vi "Find One by Column.vi"(7 "Column Criteria":refnum<class "Type.lvclass">, 8 "error in (no error)":errorcluster, 9 "Entity Definition":refnum<class "Type.lvclass">[](array[class]), 10 "Table Name":string, 11 "Database in":refnum<class "SQLite.lvclass">) -> (0 "error out":errorcluster, 2 "Result Row":refnum<class "Result Row.lvclass">, 3 "Database out":refnum<class "SQLite.lvclass">)   [LabVIEW 2020, in "Conditum SQLite.lvlib" / "SQLite.lvclass"]
uses:
  SQLite.lvclass
  SQLite.lvclass/SQLite.ctl
  <vilib>/IlluminatedG/IG Conditum Base/Conditum/Columns/Type/Type.lvclass
  <vilib>/drjdpowell/SQLite Library/SQL Connection/Connection.lvclass
  <vilib>/IlluminatedG/IG Conditum Base/Conditum/Columns/ID/ID.lvclass
  <vilib>/drjdpowell/SQLite Library/SQL Statement/SQL Statement.lvclass
  <vilib>/IlluminatedG/IG Conditum Base/Conditum/Columns/Boolean/Boolean.lvclass
  <vilib>/IlluminatedG/IG Conditum Base/Conditum/Columns/Integer/Integer.lvclass
  <vilib>/IlluminatedG/IG Conditum Base/Conditum/Columns/Double/Double.lvclass
  <vilib>/IlluminatedG/IG Conditum Base/Conditum/Columns/Timestamp/Timestamp.lvclass
  <vilib>/IlluminatedG/IG Conditum Base/Conditum/Columns/String/String.lvclass
  <vilib>/IlluminatedG/IG Conditum Base/Conditum/Database Platform/Database Platform.lvclass
  C:/Program Files (x86)/National Instruments/LabVIEW 2020/vi.lib/IlluminatedG/IG Conditum Base/Conditum/Columns/Type/Type.lvclass
  C:/Program Files (x86)/National Instruments/LabVIEW 2020/vi.lib/IlluminatedG/IG Conditum Base/Conditum/Database Platform/Database Platform.lvclass
  <vilib>/IlluminatedG/IG Conditum Base/Conditum/Result Row/Result Row.lvclass
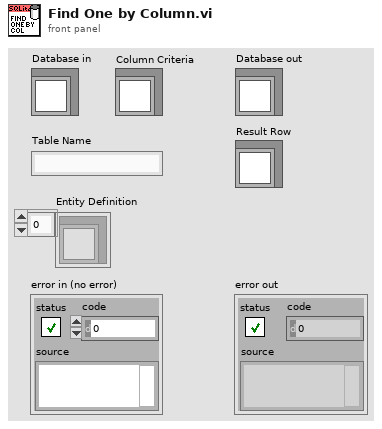
[diagram p1: front panel]
types:
  T1 = typedef "Conditum.lvlib/Field Type.ctl" = enum16{"None", "ID", "Boolean", "Integer", "Double", "Timestamp", "String", "Text", "Entity"}
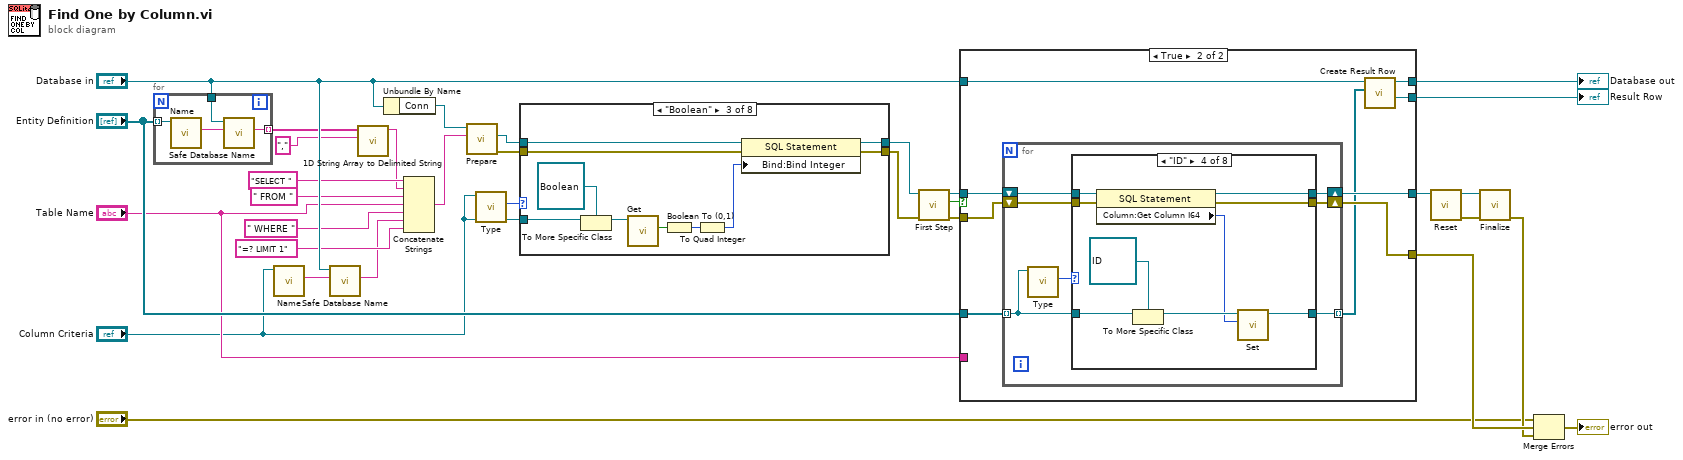
[diagram p0: block diagram]
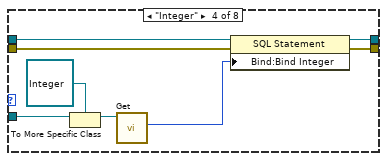
[diagram p4: hidden frame]
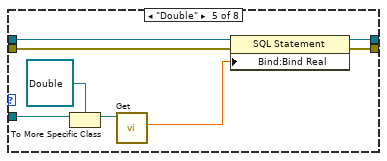
[diagram p5: hidden frame]
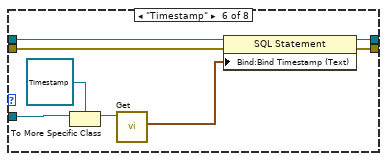
[diagram p6: hidden frame]
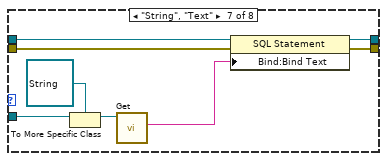
[diagram p7: hidden frame]
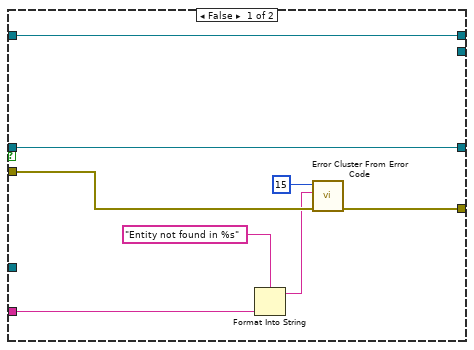
[diagram p9: hidden frame]
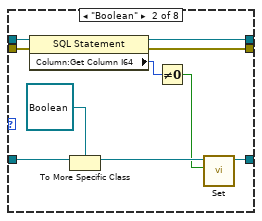
[diagram p11: hidden frame]
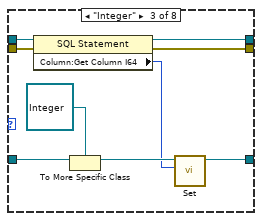
[diagram p12: hidden frame]
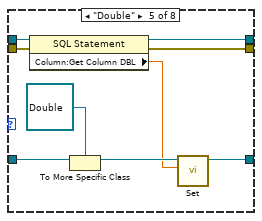
[diagram p13: hidden frame]
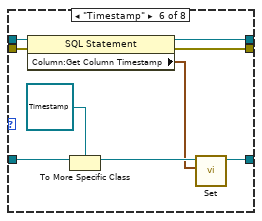
[diagram p14: hidden frame]
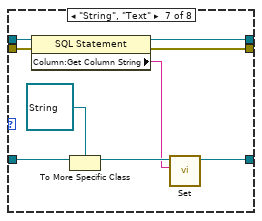
[diagram p15: hidden frame]
diagram:
  n1 = for {
    tunnel: "Entity Definition" -> [w36] mode=indexing
    tunnel: [w34] -> w30 mode=indexing
    tunnel: "Database in" -> [w33]
    n2 = call <vilib>:"Name.vi"("Type in"=w36) -> ("Table Name"=w35:string)  [unwired: 10 in]
    n3 = call-dynamic "Safe Database Name.vi"("Conditum Name"=w35, "Database in"=w33) -> ("Database Name"=w34:string)  [unwired: 9 in]
  }
  n4 = call <vilib>:"Name.vi"("Type in"="Column Criteria") -> ("Table Name"=w2:string)  [unwired: 10 in]
  n5 = call-dynamic "Safe Database Name.vi"("Conditum Name"=w2, "Database in"="Database in") -> ("Database Name"=w1:string)  [unwired: 9 in]
  n6 = call <vilib>:"1D String Array to Delimited String.vi"("delimiter"=",", "string array"=w30) -> ("delimited string"=w28:string)  [unwired: 9 in]
  n7 = Unbundle By Name("Database in") -> ("Conn"=w31:refnum<class "Connection.lvclass">)
  n8 = Concatenate Strings("SELECT ", w28, " FROM ", "Table Name", " WHERE ", w1, "=? LIMIT 1" ("string")) -> (w25:string)
  n9 = call <vilib>:"Prepare.vi"("SQL"=w25, "SQLite Connection in"=w31) -> ("error out"=w5:errorcluster, "SQL Statement"=w6:refnum<class "SQL Statement.lvclass">)  [unwired: 5 in, 3 out]
  n10 = call <vilib>:"Type.vi"("Type in"="Column Criteria") -> ("Type"=w8:T1)  [unwired: 10 in]
  n11 = case shown="\"Boolean\"" w8 {
    tunnel: w6 -> [w38 w40 w47 w55 w63 w71 w79 w84]
    tunnel: w5 -> [w37 w39 w43 w54 w62 w70 w78 w83]
    tunnel: "Column Criteria" -> [_ _ w50 w58 w66 w74 w82 _]
    tunnel: [w38 w40 w42 w53 w61 w69 w77 w84] -> w7
    tunnel: [w37 w39 w41 w52 w60 w68 w76 w83] -> w4
    frame "None", Default {
      # "#ERROR"
    }
    frame "ID" {
      # "#ERROR"
    }
    frame "Boolean" {
      n12 = To More Specific Class(target class=refnum<class "Boolean.lvclass"> refnum ("Conditum:Columns:Boolean.lvclass"), reference=w50) -> (specific class reference=w48:refnum<class "Boolean.lvclass">)  [unwired: 1 in, 1 out]
      n13 = call <vilib>:"Get.vi"("Boolean in"=w48) -> ("Value"=w46:bool)  [unwired: 10 in]
      n14 = Boolean To (0,1)(Boolean=w46) -> (0, 1=w45:i16)
      n15 = To Quad Integer(1:w45) -> (0:w44:i64)
      n16 = property class="SQL Statement"(reference=w47, error in=w43, "Bind:Bind Integer"=w44) -> (reference out=w42:refnum<class "SQL Statement.lvclass">, error out=w41:errorcluster)
    }
    frame "Integer" {
      n17 = To More Specific Class(target class=refnum<class "Integer.lvclass"> refnum ("Conditum:Columns:Integer.lvclass"), reference=w58) -> (specific class reference=w56:refnum<class "Integer.lvclass">)  [unwired: 1 in, 1 out]
      n18 = call <vilib>:"Get.vi"("Integer in"=w56) -> ("Value"=w51:i64)  [unwired: 10 in]
      n19 = property class="SQL Statement"(reference=w55, error in=w54, "Bind:Bind Integer"=w51) -> (reference out=w53:refnum<class "SQL Statement.lvclass">, error out=w52:errorcluster)
    }
    frame "Double" {
      n20 = To More Specific Class(target class=refnum<class "Double.lvclass"> refnum ("Conditum:Columns:Double.lvclass"), reference=w66) -> (specific class reference=w64:refnum<class "Double.lvclass">)  [unwired: 1 in, 1 out]
      n21 = call <vilib>:"Get.vi"("Double in"=w64) -> ("Value"=w59:dbl)  [unwired: 10 in]
      n22 = property class="SQL Statement"(reference=w63, error in=w62, "Bind:Bind Real"=w59) -> (reference out=w61:refnum<class "SQL Statement.lvclass">, error out=w60:errorcluster)
    }
    frame "Timestamp" {
      n23 = To More Specific Class(target class=refnum<class "Timestamp.lvclass"> refnum ("Conditum:Columns:Timestamp.lvclass"), reference=w74) -> (specific class reference=w72:refnum<class "Timestamp.lvclass">)  [unwired: 1 in, 1 out]
      n24 = call <vilib>:"Get.vi"("Timestamp in"=w72) -> ("Value"=w67:timestamp)  [unwired: 10 in]
      n25 = property class="SQL Statement"(reference=w71, error in=w70, "Bind:Bind Timestamp (Text)"=w67) -> (reference out=w69:refnum<class "SQL Statement.lvclass">, error out=w68:errorcluster)
    }
    frame "String", "Text" {
      n26 = To More Specific Class(target class=refnum<class "String.lvclass"> refnum ("Conditum:Columns:String.lvclass"), reference=w82) -> (specific class reference=w80:refnum<class "String.lvclass">)  [unwired: 1 in, 1 out]
      n27 = call <vilib>:"Get.vi"("String in"=w80) -> ("Value"=w75:string)  [unwired: 10 in]
      n28 = property class="SQL Statement"(reference=w79, error in=w78, "Bind:Bind Text"=w75) -> (reference out=w77:refnum<class "SQL Statement.lvclass">, error out=w76:errorcluster)
    }
    frame "Entity" {
      # "#TODO\nRelation update"
    }
  }
  n29 = call <vilib>:"First Step.vi"("error in (no error)"=w4, "SQL Statement in"=w7) -> ("error out"=w22:errorcluster, "Row returned"=w21:bool, "SQL Statement"=w23:refnum<class "SQL Statement.lvclass">)  [unwired: 7 in]
  n30 = case shown="True" w21 {
    tunnel: [w92 w101] -> w20
    tunnel: "Entity Definition" -> [_ w100]
    tunnel: "Database in" -> [w88 w99]
    tunnel: [w88 w98] -> w13
    tunnel: [_ w97] -> w12
    tunnel: w23 -> [w90 w96]
    tunnel: w22 -> [w89 w95]
    tunnel: [w90 w94] -> w19
    tunnel: "Table Name" -> [w86 _]
    frame False {
      n31 = Format Into String(format string="Entity not found in %s", w86) -> (resulting string=w85:string)  [unwired: 2 in, 1 out]
      n32 = call <vilib>:"Error Cluster From Error Code.vi"("error in (no error)"=w89, "error message (\"\")"=w85, "error code (0)"=15) -> ("error out"=w92:errorcluster)  [unwired: 6 in]
    }
    frame True {
      n33 = for {
        shift-right: [w104] -> w94
        shift-left: w96 -> [w108]
        tunnel: w100 -> [w105] mode=indexing
        tunnel: [w102] -> w93 mode=indexing
        shift-right: [w103] -> w101
        shift-left: w95 -> [w107]
        n34 = call <vilib>:"Type.vi"("Type in"=w105) -> ("Type"=w106:T1)  [unwired: 10 in]
        n35 = case shown="\"ID\"" w106 {
          tunnel: w108 -> [w110 w118 w127 w136 w145 w154 w163 w167]
          tunnel: w107 -> [w109 w117 w126 w135 w144 w153 w162 w166]
          tunnel: w105 -> [_ w120 w129 w138 w147 w156 w165 _]
          tunnel: [w110 w116 w125 w134 w143 w152 w161 w167] -> w104
          tunnel: [w109 w115 w124 w133 w142 w151 w160 w166] -> w103
          tunnel: [_ w111 w121 w130 w139 w149 w157 _] -> w102
          frame "None", Default {
            # "#ERROR"
          }
          frame "Boolean" {
            n36 = property class="SQL Statement"(reference=w118, error in=w117) -> (reference out=w116:refnum<class "SQL Statement.lvclass">, error out=w115:errorcluster, "Column:Get Column I64"=w114:i64)
            n37 = To More Specific Class(target class=refnum<class "Boolean.lvclass"> refnum ("Conditum:Columns:Boolean.lvclass"), reference=w120) -> (specific class reference=w113:refnum<class "Boolean.lvclass">)  [unwired: 1 in, 1 out]
            n38 = Not Equal To 0?(x=w114) -> (x != 0?=w112:bool)
            n39 = call <vilib>:"Set.vi"("Value"=w112, "Boolean in"=w113) -> ("Boolean out"=w111:refnum<class "Boolean.lvclass">)  [unwired: 9 in]
          }
          frame "Integer" {
            n40 = property class="SQL Statement"(reference=w127, error in=w126) -> (reference out=w125:refnum<class "SQL Statement.lvclass">, error out=w124:errorcluster, "Column:Get Column I64"=w122:i64)
            n41 = To More Specific Class(target class=refnum<class "Integer.lvclass"> refnum ("Conditum:Columns:Integer.lvclass"), reference=w129) -> (specific class reference=w123:refnum<class "Integer.lvclass">)  [unwired: 1 in, 1 out]
            n42 = call <vilib>:"Set.vi"("Value"=w122, "Integer in"=w123) -> ("Integer out"=w121:refnum<class "Integer.lvclass">)  [unwired: 9 in]
          }
          frame "ID" {
            n43 = property class="SQL Statement"(reference=w136, error in=w135) -> (reference out=w134:refnum<class "SQL Statement.lvclass">, error out=w133:errorcluster, "Column:Get Column I64"=w131:i64)
            n44 = To More Specific Class(target class=refnum<class "ID.lvclass"> refnum ("Conditum:Columns:ID.lvclass"), reference=w138) -> (specific class reference=w132:refnum<class "ID.lvclass">)  [unwired: 1 in, 1 out]
            n45 = call <vilib>:"Set.vi"("Entity ID"=w131, "ID in"=w132) -> ("ID out"=w130:refnum<class "ID.lvclass">)  [unwired: 9 in]
          }
          frame "Double" {
            n46 = property class="SQL Statement"(reference=w145, error in=w144) -> (reference out=w143:refnum<class "SQL Statement.lvclass">, error out=w142:errorcluster, "Column:Get Column DBL"=w140:dbl)
            n47 = To More Specific Class(target class=refnum<class "Double.lvclass"> refnum ("Conditum:Columns:Double.lvclass"), reference=w147) -> (specific class reference=w141:refnum<class "Double.lvclass">)  [unwired: 1 in, 1 out]
            n48 = call <vilib>:"Set.vi"("Value"=w140, "Double in"=w141) -> ("Double out"=w139:refnum<class "Double.lvclass">)  [unwired: 9 in]
          }
          frame "Timestamp" {
            n49 = property class="SQL Statement"(reference=w154, error in=w153) -> (reference out=w152:refnum<class "SQL Statement.lvclass">, error out=w151:errorcluster, "Column:Get Column Timestamp"=w148:timestamp)
            n50 = To More Specific Class(target class=refnum<class "Timestamp.lvclass"> refnum ("Conditum:Columns:Timestamp.lvclass"), reference=w156) -> (specific class reference=w150:refnum<class "Timestamp.lvclass">)  [unwired: 1 in, 1 out]
            n51 = call <vilib>:"Set.vi"("Time Stamp"=w148, "DateTime in"=w150) -> ("DateTime out"=w149:refnum<class "Timestamp.lvclass">)  [unwired: 9 in]
          }
          frame "String", "Text" {
            n52 = property class="SQL Statement"(reference=w163, error in=w162) -> (reference out=w161:refnum<class "SQL Statement.lvclass">, error out=w160:errorcluster, "Column:Get Column String"=w158:string)
            n53 = To More Specific Class(target class=refnum<class "String.lvclass"> refnum ("Conditum:Columns:String.lvclass"), reference=w165) -> (specific class reference=w159:refnum<class "String.lvclass">)  [unwired: 1 in, 1 out]
            n54 = call <vilib>:"Set.vi"("Value"=w158, "String in"=w159) -> ("String out"=w157:refnum<class "String.lvclass">)  [unwired: 9 in]
          }
          frame "Entity" {
            # "#TODO\nRelation update"
          }
        }
      }
      n55 = call <vilib>:"Create Result Row.vi"("Values"=w93, "Database in"=w99) -> ("Result"=w97:refnum<class "Result Row.lvclass">, "Database out"=w98:refnum<class "SQLite.lvclass">)  [unwired: 8 in]
    }
  }
  "Database out" <- w13
  "Result Row" <- w12
  n56 = call <vilib>:"Reset.vi"("SQL Statement in"=w19) -> ("error out"=w17:errorcluster, "SQL Statement"=w18:refnum<class "SQL Statement.lvclass">)  [unwired: 9 in]
  n57 = call <vilib>:"Finalize.vi"("error in (no error)"=w17, "SQL Statement in"=w18) -> ("error out"=w16:errorcluster)  [unwired: 9 in]
  n58 = Merge Errors("error in (no error)", w20, w16) -> (→"error out":errorcluster)
